vi "New Line to File.vi"(10 "Output File":path, 11 "Text to add":string) -> ()   [LabVIEW 2010]
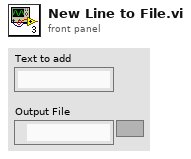
[diagram p1: front panel]
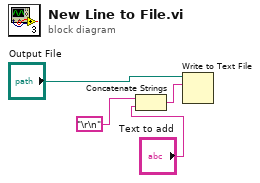
[diagram p0: block diagram]
diagram:
  n1 = Concatenate Strings("\r\n", "Text to add") -> (w1:string)
  n2 = Write to Text File(file (use dialog)="Output File", text=w1) -> ()  [unwired: 2 in, 3 out]
